vi "testrequestvariables.vi"(7 "LabVIEW Web Service Request":refnum<class "Web Request.lvclass">) -> (2 "Response":string)   [LabVIEW 2017]
uses:
  <vilib>/wsapi/Web Request.lvclass
panel:
  # "Use the Web Service Request input terminal to call the VIs on the Web Services palette. Do not remove it from the connector pane unless you don't need access to the palette."
  # "Each additional control wired to the connector pane will be available as an input in the URL. To include an indicator in terminal-mode output (the default setting), it must also be wired to the connector pane."
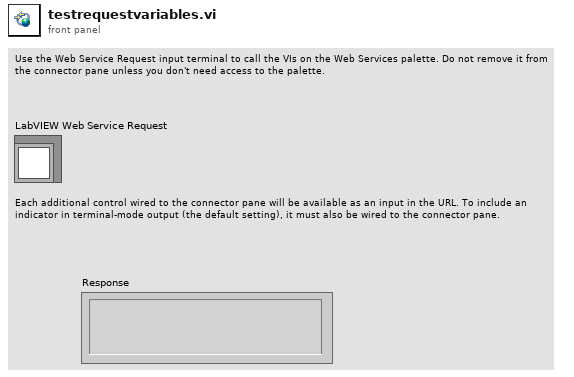
[diagram p1: front panel]
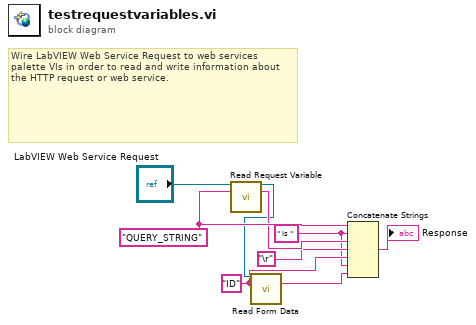
[diagram p0: block diagram]
diagram:
  w3 = "ID" ("key")
  w2 = " is " ("string")
  w8 = "QUERY_STRING" ("variable name")
  # "Wire LabVIEW Web Service Request to web services palette VIs in order to read and write information about the HTTP request or web service."
  n1 = call <vilib>:"Read Request Variable.vi"("LabVIEW Web Service Request"="LabVIEW Web Service Request", "variable name"=w8) -> ("LabVIEW Web Service Request out"=w5:refnum<class "Web Request.lvclass">, "value"=w7:string)  [unwired: 11 in, 1 out]
  n2 = call <vilib>:"Read Form Data.vi"("LabVIEW Web Service Request"=w5, "key"=w3) -> ("value"=w1:string)  [unwired: 10 in, 3 out]
  n3 = Concatenate Strings(w8, w2, w7, "\r", w3, w2, w1) -> (→"Response":string)
